vi "vehicle suspension final.vi"() -> ()   [LabVIEW 2012]
uses:
  <vilib>/addons/control/pid/pid.llb/PID (DBL).vi
  <vilib>/imath/engines/lvmath2/RunTimeEngine/NodeEndStatement/NIMS_NodeEndStatement_Output.vi
  <instcachedir>/0/NIMS_NodeEndStatement_Output_53EC0D466D134D7ABD903AC30B43404B.lvgen/NIMS_NodeEndStatement_Output_53EC0D466D134D7ABD903AC30B43404B_010.vi
  <vilib>/imath/engines/lvmath2/RunTimeEngine/ErrorHandling/NIMS_Finalize Error.vi
  <vilib>/express/express arith-compare/Formula/XNode/ExpressFormulaBlockNode.xnode
  <vilib>/addons/control/pid/NI_PID_pid.lvlib
panel:
  in  "stop":bool
  in  "Vehicle Parameters":T1
  out "f2":cdb
  out "f1":cdb
  in  "Disturbance Inp(W)":dbl format="%.2f"
  out "Z2":dbl(graph)
  out "Z2 dot":dbl format="%.2f"
  out "Z1":dbl(graph)
  out "Z1 dot":dbl format="%.2f"
  out "Z1-Z2":dbl(graph)
  out "(Z1-Z2)dot":dbl format="%.2f"
  in  "Control Input(U)":dbl
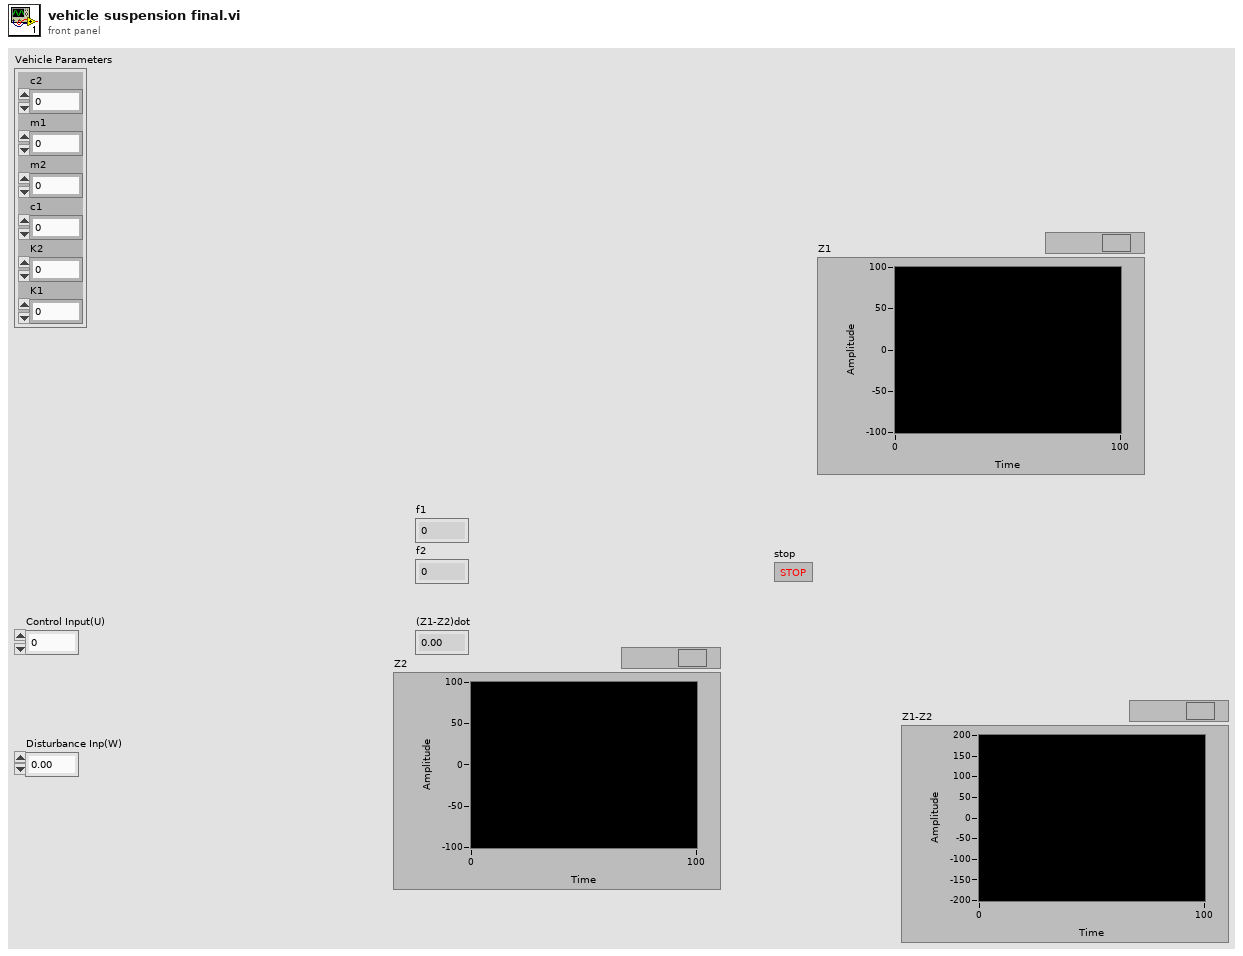
[diagram p1: front panel]
types:
  T1 = cluster{"c2":i32, "m1":i32, "m2":i32, "c1":i32, "K2":i32, "K1":i32}
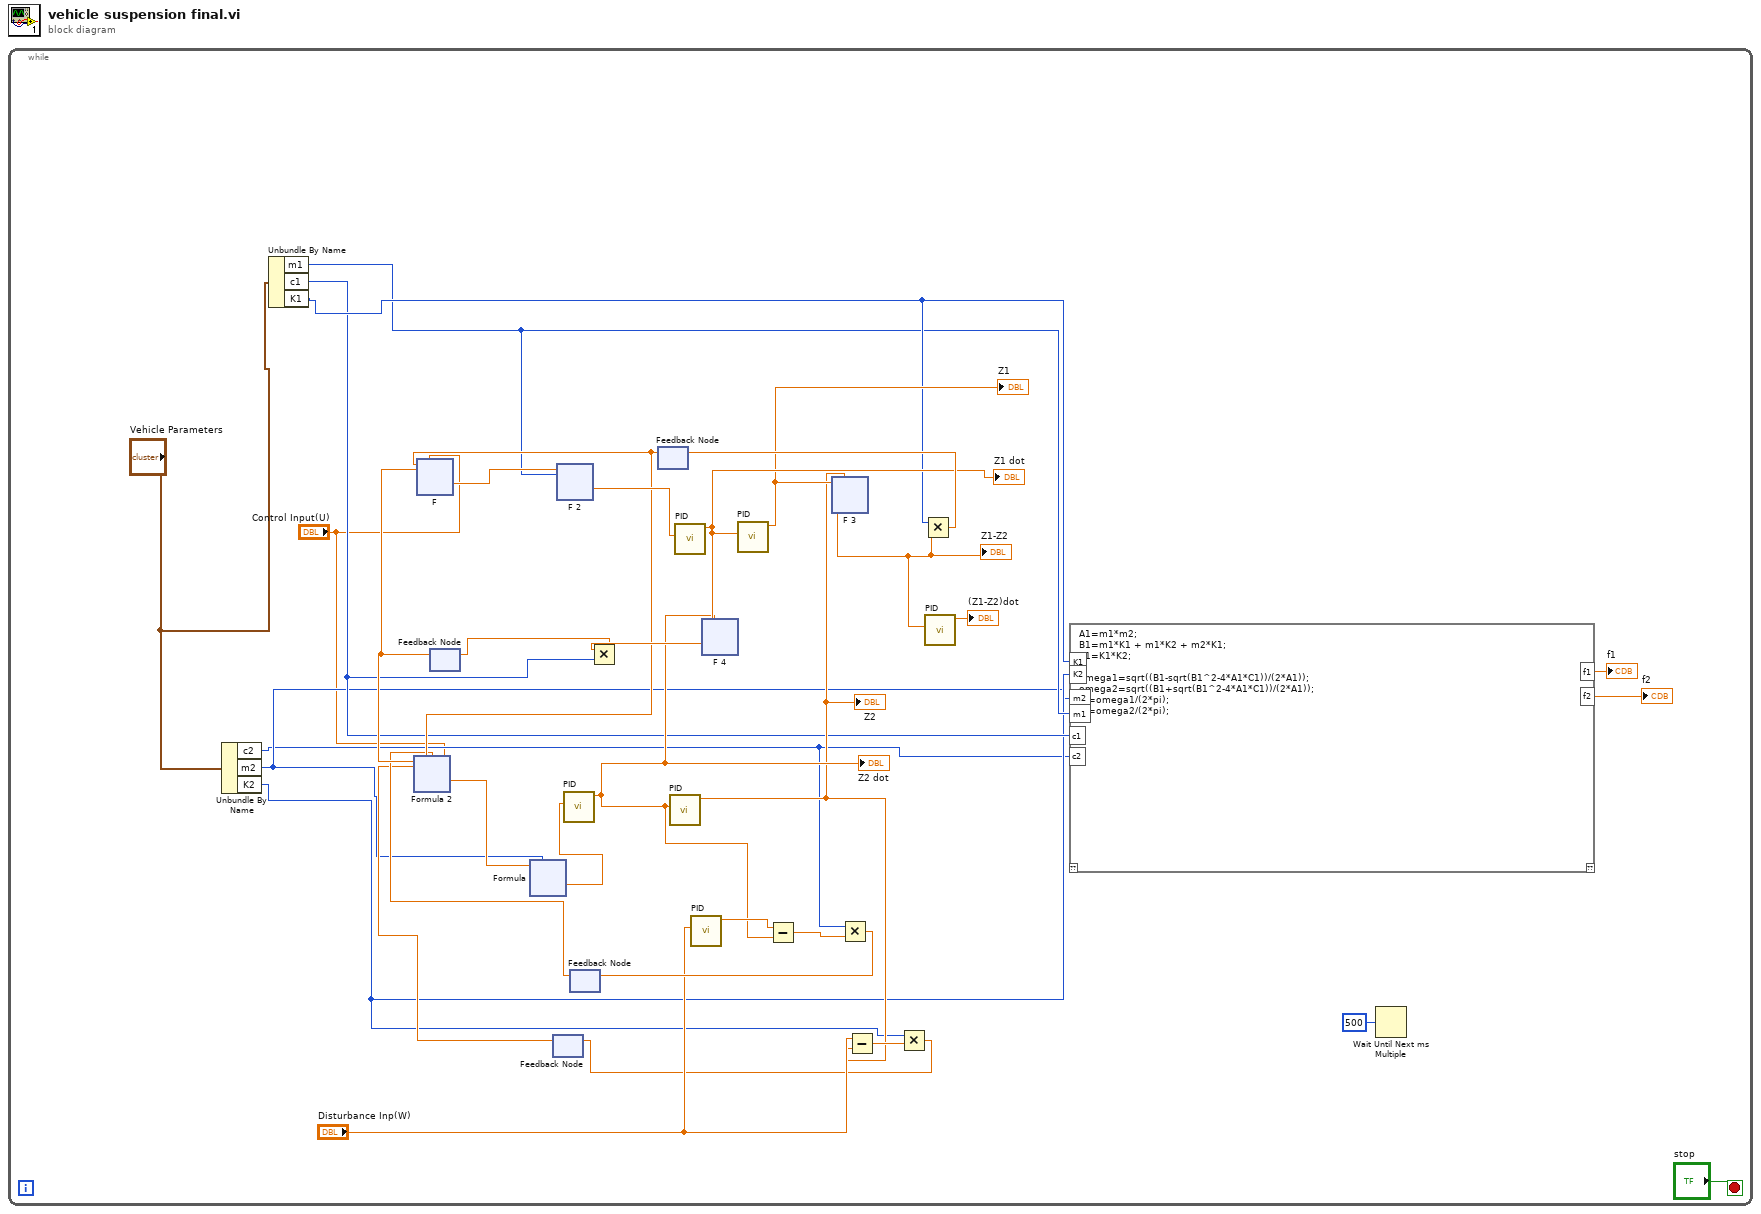
[diagram p0: block diagram]
diagram:
  n1 = while {
    stop <- "stop" stop-if-true
    n2 = Unbundle By Name("Vehicle Parameters") -> ("c2"=w5:i32, "m2"=w6:i32, "K2"=w7:i32)
    n3 = Unbundle By Name("Vehicle Parameters") -> ("m1"=w9:i32, "c1"=w8:i32, "K1"=w10:i32)
    n4 = feedback #1() -> (w27:dbl)  [unwired: 1 in]
    n5 = feedback #2() -> (w15:dbl)  [unwired: 1 in]
    n6 = feedback #3() -> (w19:dbl)  [unwired: 1 in]
    n7 = feedback #4() -> (w26:dbl)  [unwired: 1 in]
    n8 = xnode "Formula 2"("X1"=w27, "X2"=w26, "X3"=w19, "X4"=w15, "X5"="Control Input(U)") -> ("Result"=w25:dbl)  [unwired: 1 in, 1 out]
    n9 = xnode "F"("X1"=w26, "U"="Control Input(U)", "X3"=w27) -> ("Result"=w34:dbl)  [unwired: 1 in, 1 out]
    n10 = xnode "Formula"("X1"=w25, "X2"=w6) -> ("Result"=w24:dbl)  [unwired: 1 in, 1 out]
    n11 = xnode "F 2"("Out"=w34, "m1"=w9) -> ("Result"=w35:dbl)  [unwired: 1 in, 1 out]
    n12 = call-poly <vilib>:"PID.vi"("process variable"=w24) -> ("output"=w22:dbl)  [unwired: 9 in, 1 out]
    "Z2 dot" <- w22
    n13 = call-poly <vilib>:"PID.vi"("process variable"=w22) -> ("output"=w11:dbl)  [unwired: 9 in, 1 out]
    "Z2" <- w11
    n14 = call-poly <vilib>:"PID.vi"("process variable"=w35) -> ("output"=w30:dbl)  [unwired: 9 in, 1 out]
    "Z1 dot" <- w30
    n15 = call-poly <vilib>:"PID.vi"("process variable"="Disturbance Inp(W)") -> ("output"=w23:dbl)  [unwired: 9 in, 1 out]
    n16 = xnode "F 4"("Z1_dot"=w30, "Z2_dot"=w22) -> ("Result"=w29:dbl)  [unwired: 1 in, 1 out]
    n17 = Multiply(x=w29, y=w8) -> (x*y=w28:dbl)
    n18 = feedback-in #1(w28) -> ()
    n19 = call-poly <vilib>:"PID.vi"("process variable"=w30) -> ("output"=w12:dbl)  [unwired: 9 in, 1 out]
    "Z1" <- w12
    n20 = Subtract(x=w23, y=w22) -> (x-y=w21:dbl)
    n21 = xnode "F 3"("Z1"=w12, "Z2"=w11) -> ("Result"=w32:dbl)  [unwired: 1 in, 1 out]
    "Z1-Z2" <- w32
    n22 = Multiply(x=w5, y=w21) -> (x*y=w20:dbl)
    n23 = feedback-in #3(w20) -> ()
    n24 = Subtract(x="Disturbance Inp(W)", y=w11) -> (x-y=w17:dbl)
    n25 = Multiply(x=w7, y=w17) -> (x*y=w16:dbl)
    n26 = feedback-in #2(w16) -> ()
    n27 = Multiply(x=w10, y=w32) -> (x*y=w33:dbl)
    n28 = feedback-in #4(w33) -> ()
    n29 = call-poly <vilib>:"PID.vi"("process variable"=w32) -> ("output"=→"(Z1-Z2)dot":dbl)  [unwired: 9 in, 1 out]
    n30 = mathscript code="A1=m1*m2;\nB1=m1*K1 + m1*K2 + m2*K1;\nC1=K1*K2;\n\nomega1=sqrt((B1-sqrt(B1^2-4*A1*C1))/(2*A1));\nomega2=sqrt((B1+sqrt(B1^2-4*A1*C1))/(2*A1));\nf1=omega1/(2*pi);\nf2=omega2/(2*pi);"("K1"=w10, "K2"=w7, "m2"=w6, "m1"=w9, "c1"=w8, "c2"=w5) -> ("f1"=→"f1":cdb, "f2"=→"f2":cdb)  [unwired: 1 in, 1 out]
    n31 = Wait Until Next ms Multiple(millisecond multiple=u32 500) -> ()  [unwired: 1 out]
  }
